vi "getChannelConfig.vi"(8 "error in":T1, 11 "Channel":i32) -> (0 "error out":T2, 1 "Averaging?":bool, 2 "source":i32, 3 "trigger":i32, 5 "smpTime":dbl format="%#_g s")   [LabVIEW 2016]
doc: "Reads out the channel configuration. The paramters are\n-Channel: Number of the channel of interest (0 to 13)\n-Trigger: Trigger source for data output\n-Source: Data source for the channel\n-Averaging?: If data is averaged over the sample time\n-smpTime: Time per sample in seconds."
uses:
  Controls/Error_Out.ctl
  Controls/Error_In.ctl
  Files_ASC500/DLL/daisybase.dll
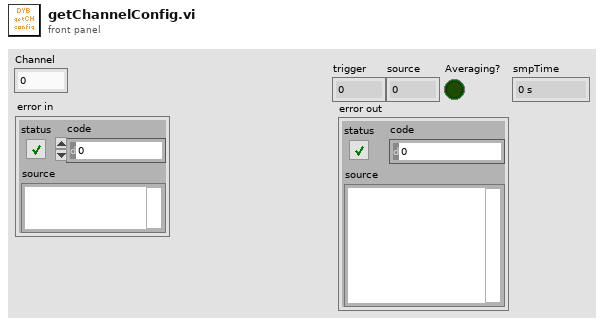
[diagram p1: front panel]
types:
  T1 = typedef "Error_In.ctl" = errorcluster
  T2 = typedef "Error_Out.ctl" = errorcluster
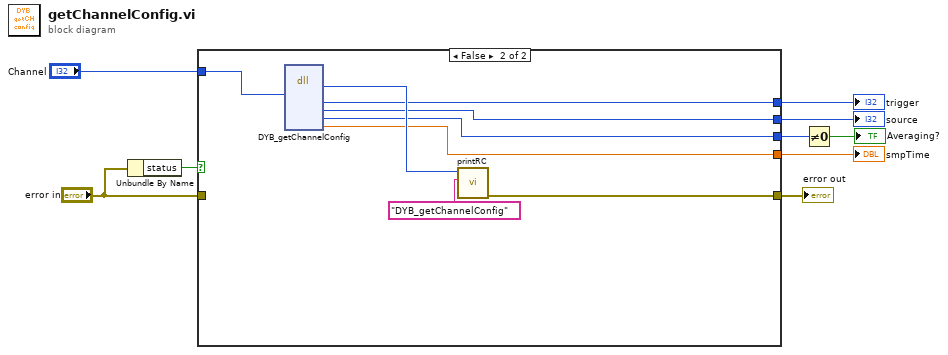
[diagram p0: block diagram]
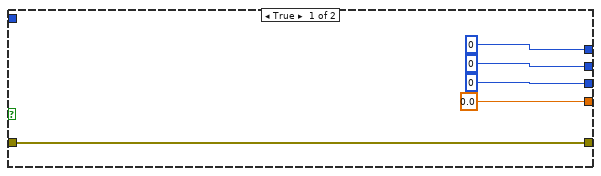
[diagram p2: hidden frame]
diagram:
  n1 = Unbundle By Name("error in") -> ("status"=w9:bool)
  n2 = case shown="False" w9 {
    tunnel: [w14 w20] -> w7
    tunnel: "Channel" -> [_ w22]
    tunnel: "error in" -> [w14 _]
    tunnel: [0 w19] -> w5
    tunnel: [0 w18] -> w4
    tunnel: [i16 0 w17] -> w2
    tunnel: [0.0 w15] -> w3
    frame True {
    }
    frame False {
      n3 = dll-call lib="G:/SCMOperations/Share/ELE/Produkt Information/ASC500/04 Remote Control/02 development versions/2018Nov06/Files_ASC500/DLL/daisybase.dll" fn="DYB_getChannelConfig"("Channel"=w22) -> ("return code"=w21:i32, "trigger"=w19:i32, "source"=w18:i32, "average"=w17:u32, "smpTime"=w15:dbl)  [unwired: 8 in, 2 out]
      n4 = call "printRC.vi"("additional information"="DYB_getChannelConfig", "RC"=w21) -> ("error out"=w20:T2)  [unwired: 9 in]
    }
  }
  "error out" <- w7
  "trigger" <- w5
  "source" <- w4
  "smpTime" <- w3
  n5 = Not Equal To 0?(x=w2) -> (x != 0?=→"Averaging?":bool)
